vi "Day 3.vi"() -> ()   [LabVIEW 2019]
panel:
  out "Non-Overlapping Elf Claim":i32
  out "in^2 of Overlapping Claims":i32
  out "Trimmed Array":string[](array[string])
  out "Error Out":errorcluster
  out "1D String Array":string[](array[string])
  in  "Error In":errorcluster
  in  "Relative Path to Input File":string
  # "Part 1"
  # "Part 2"
  # "I have a python script that I stole...\nSecond answer is 909"
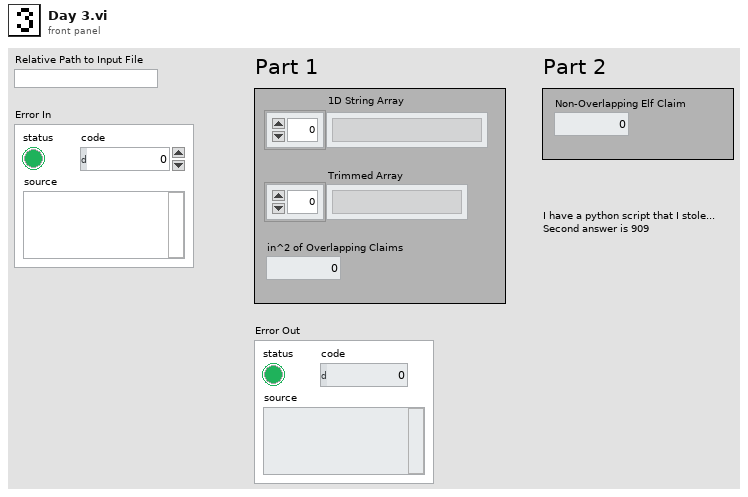
[diagram p1: front panel]
types:
  T1 = typedef "Real Matrix NI_Silver.ctl" = dbl[][]
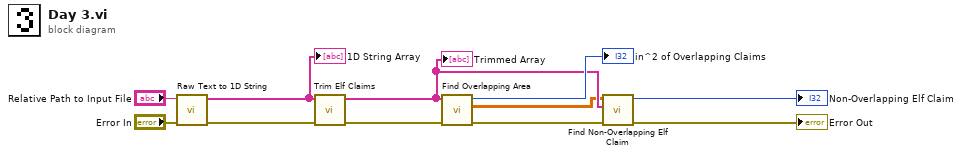
[diagram p0: block diagram]
diagram:
  n1 = call "Raw Text to 1D String.vi"("Error In"="Error In", "Relative Path to Input File"="Relative Path to Input File") -> ("Error Out"=w8:errorcluster, "1D String Array"=w9:string[])  [unwired: 8 in]
  "1D String Array" <- w9
  n2 = call "Trim Elf Claims.vi"("error in (no error)"=w8, "1D String Array"=w9) -> ("error out"=w6:errorcluster, "Trimmed Array"=w5:string[])  [unwired: 8 in]
  "Trimmed Array" <- w5
  n3 = call "Find Overlapping Area.vi"("Error In"=w6, "List of Trimmed Claims"=w5) -> ("Error Out"=w2:errorcluster, "Fabric Claims"=w4:T1, "in^2 of Overlapping Claims"=→"in^2 of Overlapping Claims":i32)  [unwired: 7 in]
  n4 = call "Find Non-Overlapping Elf Claim.vi"("error in (no error)"=w2, "Trimmed Array"=w5, "Fabric Claims"=w4) -> ("error out"=→"Error Out":errorcluster, "Non-Overlapping Elf Claim"=→"Non-Overlapping Elf Claim":i32)  [unwired: 7 in]
